vi "Invoke_node2Practice.vi"() -> ()   [LabVIEW 2019]
panel:
  in  "stop":bool
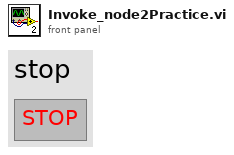
[diagram p1: front panel]
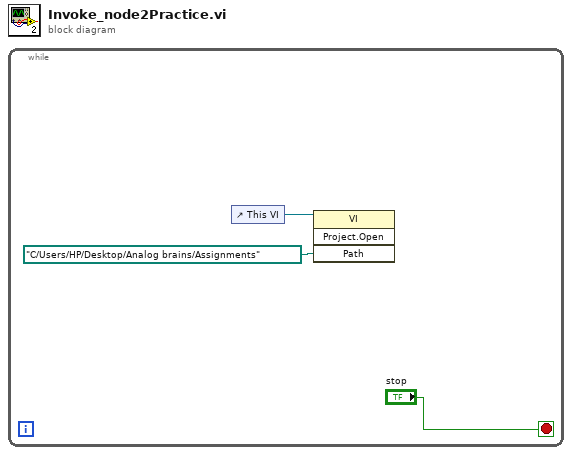
[diagram p0: block diagram]
diagram:
  n1 = while {
    stop <- "stop" stop-if-true
    n2 = control-ref of="This VI"() -> (w2:refnum<vi>)
    n3 = invoke class="VI" method="Project.Open"(reference=w2, "Path"=path "C:/Users/HP/Desktop/Analog brains/Assignments") -> ()  [unwired: 2 in, 4 out]
  }
